vi "Generate Cartesian Trajectory (Array).vi"(7 "intermediate points":dbl[](array[numeric]), 8 "error in (no error)":errorcluster, 10 "end transform":T1, 11 "start transform":T1) -> (0 "error out":errorcluster, 3 "interpolated trajectory":dbl[][][](array[numeric]))   [LabVIEW 2017, in "NI_Kinematics.lvlib"]
doc: "Generates a smooth trajectory of end effector positions between two points in Cartesian space. Wire data to the <B>intermediate points</B> input to determine the polymorphic instance to use or manually select the instance.\n\n<B>.m file:</B> ctraj"
uses:
  <vilib>/robotics/Kinematics/NI_Kinematics.lvlib
  <vilib>/Analysis/Matrix/Datatypes/RealMatrix.ctl
  <vilib>/robotics/Kinematics/Rotation Matrix to Quaternion.vi
  <vilib>/robotics/Kinematics/Get Translation Vector.vi
  <vilib>/robotics/Kinematics/Rotation Matrix to Transform.vi
  <vilib>/robotics/Kinematics/Interpolate Quaternions.vi
  <vilib>/robotics/Kinematics/Quaternion to Rotation Matrix.vi
  <vilib>/robotics/Utilities/Generate Error.vi
  <vilib>/Analysis/baseanly.llb/Dot Product.vi
  <vilib>/Analysis/baseanly.llb/Real Dot Product.vi
  <vilib>/Analysis/baseanly.llb/Outer Product.vi
  <vilib>/Analysis/baseanly.llb/Real Outer Product.vi
  <vilib>/robotics/Kinematics/Create Lie Group Matrix.vi
  <vilib>/Analysis/Matrix/Numeric/Add/Add.vi
  <vilib>/Analysis/Matrix/Numeric/Add/Add - RM,RM.vi
  <vilib>/Analysis/Matrix/Numeric/Multiply/Multiply.vi
  <vilib>/Analysis/Matrix/Numeric/Multiply/Multiply - RM,R.vi
  <vilib>/Analysis/Matrix/Numeric/Multiply/Multiply - R,RM.vi
  <vilib>/robotics/Kinematics/Rotation Matrix to Angle Vector.vi
  <vilib>/Analysis/Matrix/NI_Matrix.lvlib
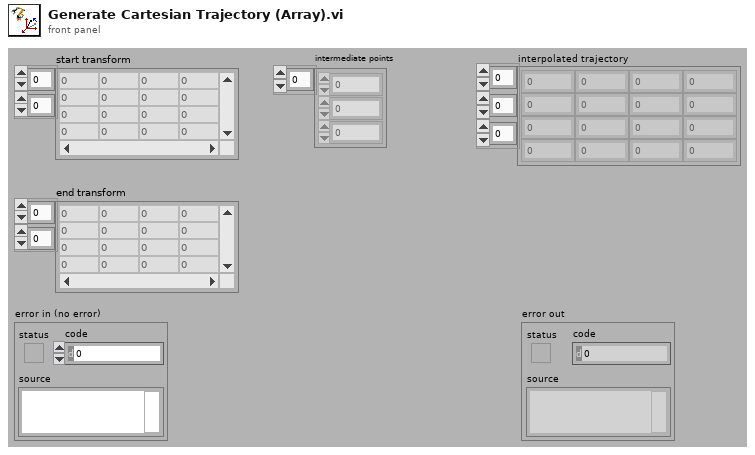
[diagram p1: front panel]
types:
  T1 = typedef "NI_Matrix.lvlib/RealMatrix.ctl" = dbl[][]
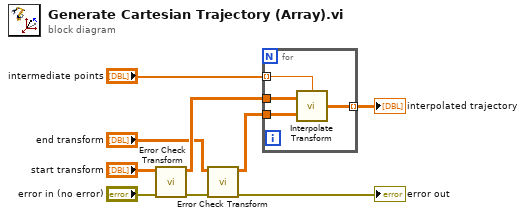
[diagram p0: block diagram]
diagram:
  n1 = call <vilib>:"Error Check Transform.vi"("error in (no error)"="error in (no error)", "Transform in"="start transform") -> ("error out"=w3:errorcluster, "Transform out"=w6:T1)  [unwired: 8 in]
  n2 = call <vilib>:"Error Check Transform.vi"("error in (no error)"=w3, "Transform in"="end transform") -> ("error out"=→"error out":errorcluster, "Transform out"=w4:T1)  [unwired: 8 in]
  n3 = for {
    tunnel: "intermediate points" -> [w13] mode=indexing
    tunnel: w6 -> [w12]
    tunnel: w4 -> [w11]
    tunnel: [w10] -> w8 mode=indexing
    n4 = call <vilib>:"Interpolate Transform.vi"("r"=w13, "transform 2"=w11, "transform 1"=w12) -> ("interpolation"=w10:T1)
  }
  "interpolated trajectory" <- w8
